vi "Tosca-Get Pretrial Property Table (vi).vi"(0 "Path":path, 11 "error in (no error)":errorcluster) -> (8 "Table":T1[](array[typedef]), 15 "error out":errorcluster)   [LabVIEW 2020]
uses:
  epl-vi-lib/Utility VIs/Controls/KPropertyTable/RowData.ctl
  epl-vi-lib/Utility VIs/Controls/KPropertyTable/DataType.ctl
  epl-vi-lib/Utility VIs/Controls/KPropertyTable/KPropertyTable.xctl
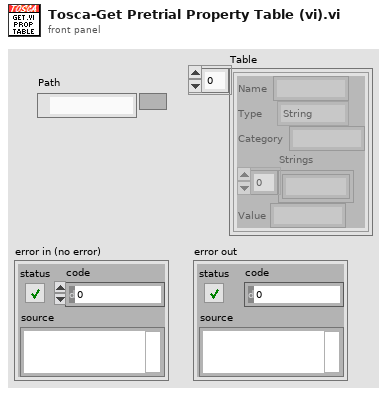
[diagram p1: front panel]
types:
  T1 = typedef "KPropertyTable.xctl/RowData.ctl" = cluster{"Name":string, "Type":T2, "Category":string, "Strings":string[], "Value":string}
  T2 = typedef "KPropertyTable.xctl/DataType.ctl" = enum16{"String", "Enum", "Int", "Double", "Boolean", "Ring", "Formula"}
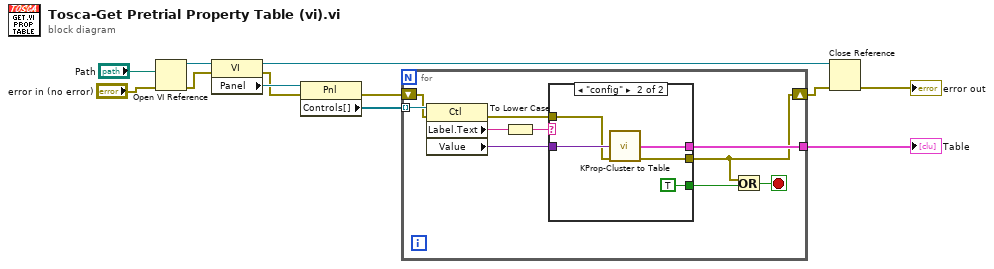
[diagram p0: block diagram]
diagram:
  n1 = Open VI Reference(vi path="Path", error in (no error)="error in (no error)") -> (vi reference=w10:refnum<vi>, error out=w9:errorcluster)  [unwired: 4 in]
  n2 = property class="VI"(reference=w10, error in=w9) -> (reference out=w1:refnum<vi>, error out=w7:errorcluster, "Panel"=w8:refnum<vi>)
  n3 = property class="Pnl"(reference=w8, error in=w7) -> (error out=w5:errorcluster, "Controls[]"=w6:refnum<vi>[])  [unwired: 1 out]
  n4 = for {
    tunnel: w6 -> [w22] mode=indexing
    shift-right: [w14] -> w3
    shift-left: w5 -> [w19]
    tunnel: [w16] -> w4
    stop <- w15 stop-if-true
    n5 = property class="Ctl"(reference=w22, error in=w19) -> (error out=w17:errorcluster, "Label.Text"=w21:string, "Value"=w18:variant)  [unwired: 1 out]
    n6 = To Lower Case(string=w21) -> (all lower case string=w20:string)
    n7 = case shown="\"config\"" w20 {
      tunnel: w18 -> [_ w28]
      tunnel: w17 -> [w23 w27]
      tunnel: [_ w26] -> w16
      tunnel: [w23 w25] -> w14
      tunnel: [_ TRUE] -> w13
      frame "", Default {
      }
      frame "config" {
        n8 = call "KProp-Cluster to Table.vi"("Anything"=w28, "Error In"=w27) -> ("Rows"=w26:T1[], "Error Out"=w25:errorcluster)  [unwired: 12 in]
      }
    }
    n9 = Or(x=w14, y=w13) -> (x .or. y?=w15:bool)
  }
  "Table" <- w4
  n10 = Close Reference(reference=w1, error in (no error)=w3) -> (error out=→"error out":errorcluster)
